vi "FTW-JSON-SerializeElement.vi"(0 "JSON Object":refnum<data-value>, 5 "Key":string, 11 "error in":errorcluster) -> (4 "JSON Object out":refnum<data-value>, 6 "Element as JSON String":string, 10 "Found?":bool, 15 "error out":errorcluster)   [LabVIEW 2015]
uses:
  core/FTW-JSON-Core-Structure.ctl
panel:
  # "Inputs"
  # "Outputs"
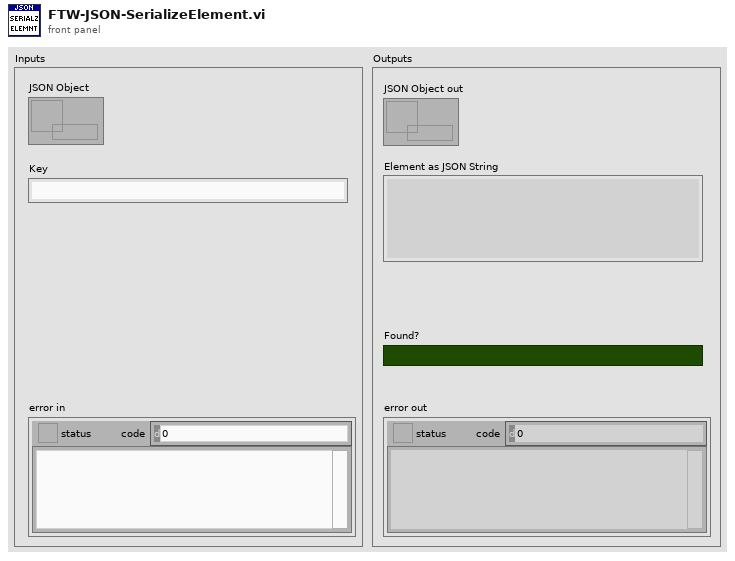
[diagram p1: front panel]
types:
  T1 = typedef "FTW-JSON-Core-Structure.ctl" = cluster{"JSON Object":i64, "Encoding Flags":i64, "Decoding Flags":i64}
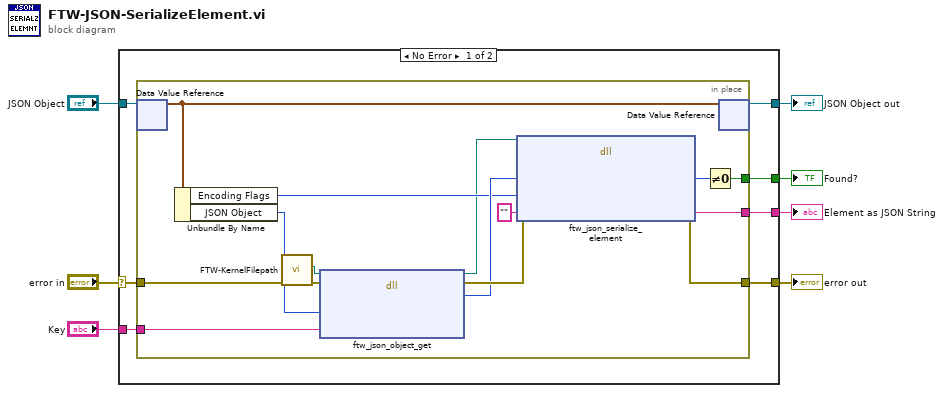
[diagram p0: block diagram]
diagram:
  n1 = case shown="No Error" "error in" {
    selector: "error in" -> [w14 w31]
    tunnel: [w11 w31] -> w7
    tunnel: [w8 w30] -> w5
    tunnel: "JSON Object" -> [w9 w30]
    tunnel: "Key" -> [w13 _]
    tunnel: [w12 _] -> w2
    tunnel: [w10 _] -> w1
    frame No Error {
      n2 = in-place {
        in-place-border: w14 -> [w18]
        in-place-border: w13 -> [w29]
        in-place-border: [w28] -> w12
        in-place-border: [w20] -> w11
        in-place-border: [w23] -> w10
        n3 = in-place-dvr #1(w9) -> (w26:T1)  [unwired: 1 out]
        n4 = Unbundle By Name(w26) -> ("Encoding Flags"=w21:i64, "JSON Object"=w27:i64)
        n5 = call "FTW-KernelFilepath.vi"("error in"=w18) -> ("error out"=w17:errorcluster, "Library Filepath"=w16:path)  [unwired: 8 in, 1 out]
        n6 = dll-call lib="?" fn="ftw_json_object_get"(path in=w16, error in=w17, "JSON Object Pointer"=w27, "Element Key"=w29) -> (path out=w15:path, error out=w24:errorcluster, "JSON Element Pointer"=w22:i64)  [unwired: 3 in]
        n7 = dll-call lib="?" fn="ftw_json_serialize_element"(path in=w15, error in=w24, "JSON Object Pointer"=w22, "Flags"=w21, "Serialized String"="") -> (error out=w20:errorcluster, "JSON Object Pointer"=w19:i64, "Serialized String"=w23:string)  [unwired: 3 in, 1 out]
        n8 = Not Equal To 0?(x=w19) -> (x != 0?=w28:bool)
        n9 = in-place-dvr #1(w26) -> (w8:refnum<data-value>)  [unwired: 1 out]
      }
    }
    frame Error {
    }
  }
  "error out" <- w7
  "JSON Object out" <- w5
  "Found?" <- w2
  "Element as JSON String" <- w1
